vi "固定站质控流程参数读取对话框.vi"(11 "标题":string="质控流程读写") -> ()   [LabVIEW 2016, in "质控单元.lvlib"]
uses:
  <vilib>/Utility/miscctls.llb/LVPointTypeDef.ctl
panel:
  out "流程写入U16":u16[](array[numeric])
  out "退出中间":bool=TRUE
  in  "站号":enum16{"", "氨氮", "总磷", "总氮", "CODMn", "CODCr"}(ring)
  out "排液流程":u16[](array[numeric])
  out "加标流程":u16[](array[numeric])
  out "水样流程":u16[](array[numeric])
  in  "流程保存到电脑":bool
  in  "从电脑读取流程":bool
  in  "步骤10枚举":enum16{"加标", "进样", "排液", "搅拌", "定量"}(ring)
  in  "步骤10参数":dbl
  in  "步骤9枚举":enum16{"加标", "进样", "排液", "搅拌", "定量"}(ring)
  in  "步骤9参数":dbl
  in  "步骤8枚举":enum16{"加标", "进样", "排液", "搅拌", "定量"}(ring)
  in  "步骤8参数":dbl
  in  "步骤7枚举":enum16{"加标", "进样", "排液", "搅拌", "定量"}(ring)
  in  "步骤7参数":dbl
  in  "步骤6枚举":enum16{"加标", "进样", "排液", "搅拌", "定量"}(ring)
  in  "步骤6参数":dbl
  in  "步骤5枚举":enum16{"加标", "进样", "排液", "搅拌", "定量"}(ring)
  in  "步骤5参数":dbl
  in  "步骤4枚举":enum16{"加标", "进样", "排液", "搅拌", "定量"}(ring)
  in  "步骤4参数":dbl
  in  "步骤3枚举":enum16{"加标", "进样", "排液", "搅拌", "定量"}(ring)
  in  "步骤3参数":dbl
  in  "步骤2枚举":enum16{"加标", "进样", "排液", "搅拌", "定量"}(ring)
  in  "步骤2参数":dbl
  in  "步骤1枚举":enum16{"加标", "进样", "排液", "搅拌", "定量"}(ring)
  in  "步骤1参数":dbl
  in  "小流程":u16(ring) items=["润洗", "进样"]
  in  "大流程":enum16{"水样流程", "加标流程", "排液流程"}(ring)
  in  "退出":bool
  in  "流程写入到设备":bool
  in  "从设备读取流程":bool
  # "步骤1"
  # "秒/毫升"
  # "步骤2"
  # "秒/毫升"
  # "步骤3"
  # "秒/毫升"
  # "步骤4"
  # "秒/毫升"
  # "步骤5"
  # "秒/毫升"
  # "步骤6"
  # "秒/毫升"
  # "步骤7"
  # "秒/毫升"
  # "步骤8"
  # "秒/毫升"
  # "步骤9"
  # "秒/毫升"
  # "步骤10"
  # "秒/毫升"
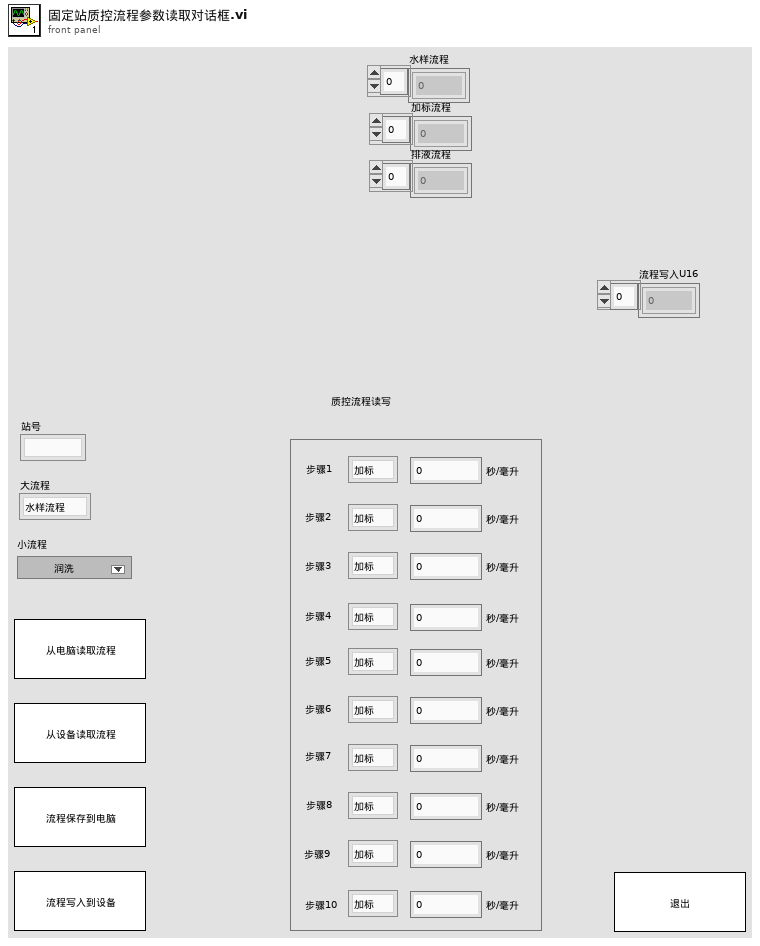
[diagram p1: front panel]
types:
  T1 = typedef "LVPointTypeDef.ctl" = cluster{"Horizontal":i16, "Vertical":i16}
  T2 = cluster{"flow1":cluster{"Type":u16, "Value":sgl}[], "flow2":cluster{"Type":u16, "Value":sgl}[], "flow3":cluster{"Type":u16, "Value":sgl}[]}
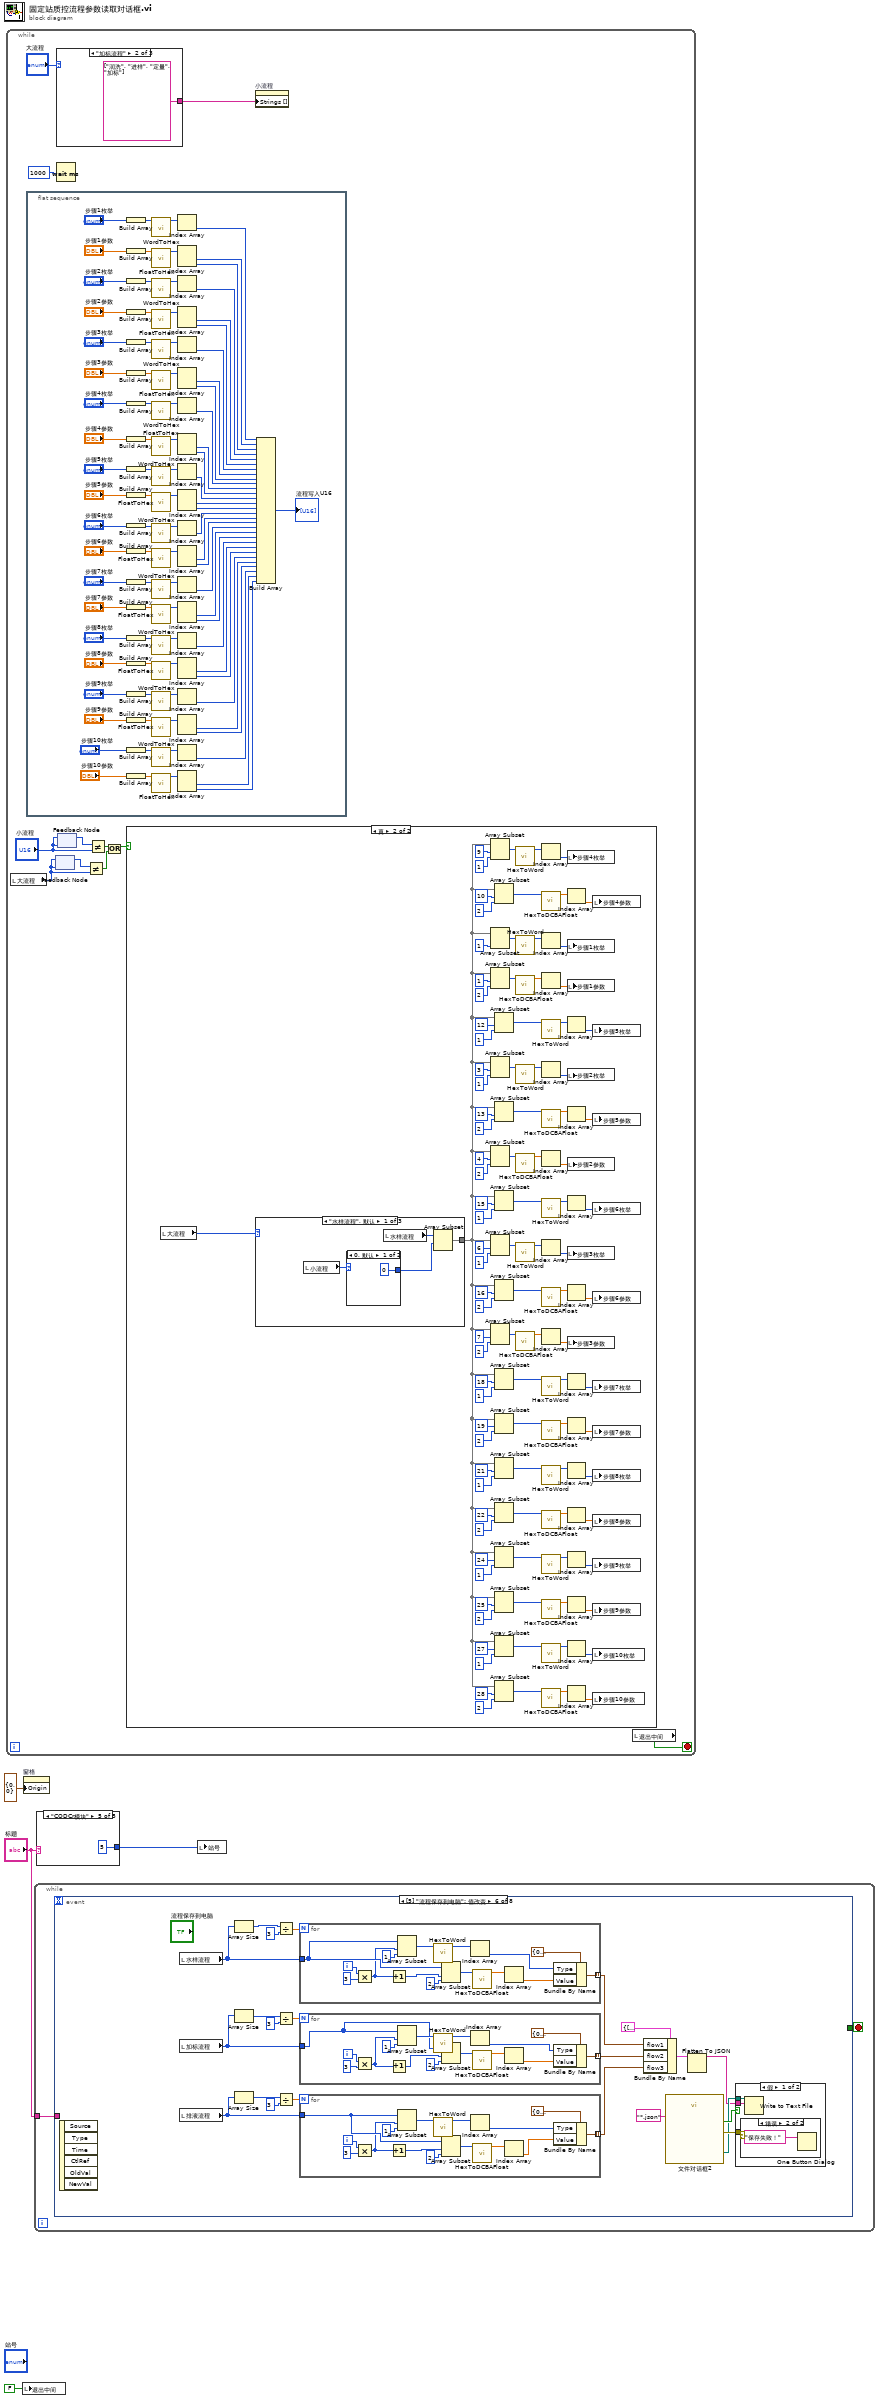
[diagram p0: block diagram]
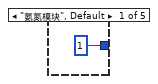
[diagram p2: hidden frame]
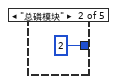
[diagram p3: hidden frame]
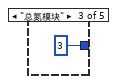
[diagram p4: hidden frame]
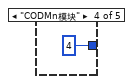
[diagram p5: hidden frame]
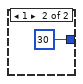
[diagram p7: hidden frame]
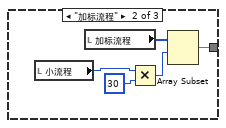
[diagram p8: hidden frame]
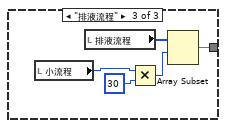
[diagram p9: hidden frame]
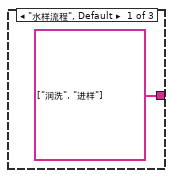
[diagram p10: hidden frame]
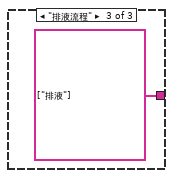
[diagram p11: hidden frame]
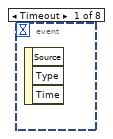
[diagram p12: hidden frame]
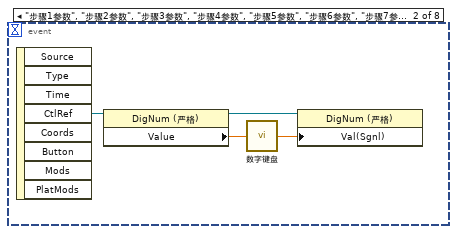
[diagram p13: hidden frame]
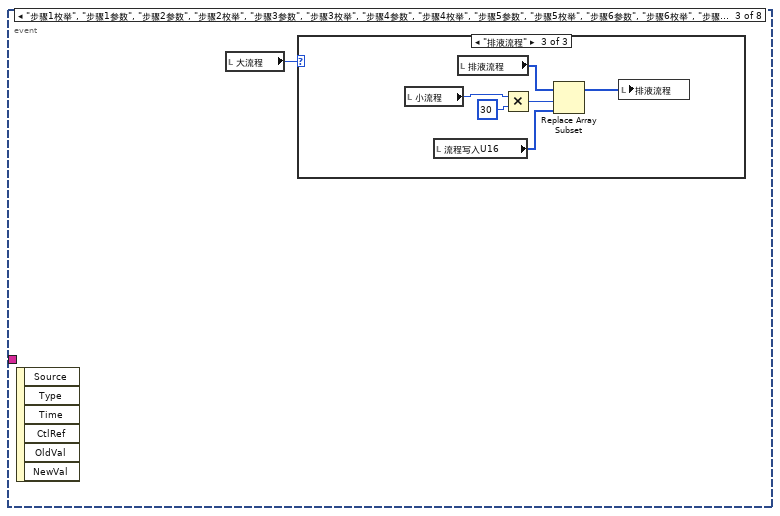
[diagram p14: hidden frame]
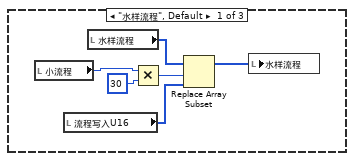
[diagram p15: hidden frame]
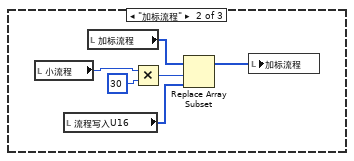
[diagram p16: hidden frame]
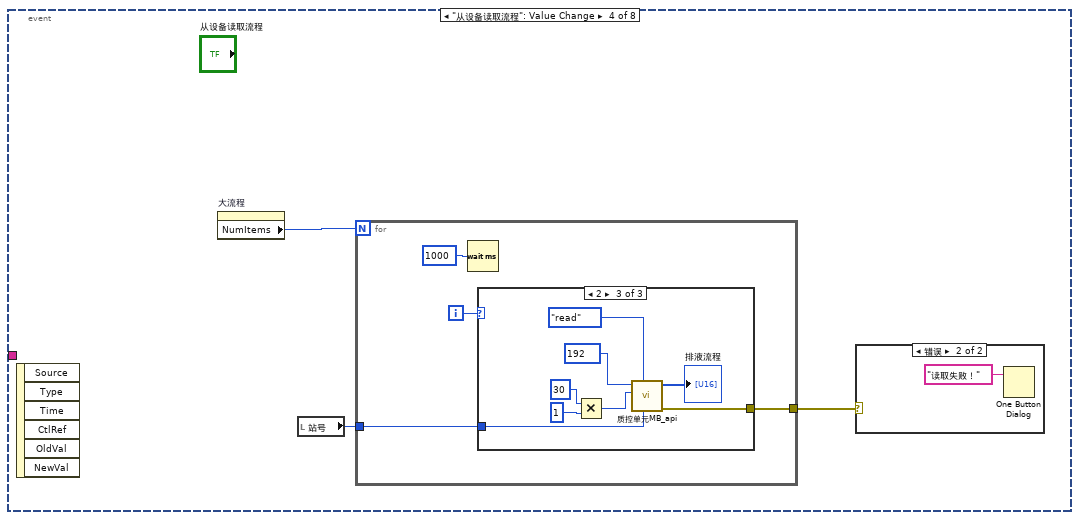
[diagram p17: hidden frame]
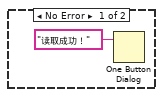
[diagram p18: hidden frame]
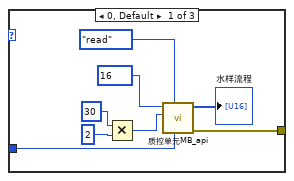
[diagram p19: hidden frame]
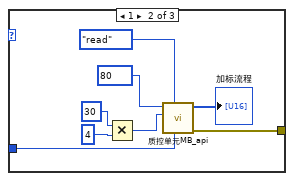
[diagram p20: hidden frame]
diagram:
  n1 = while {
    stop <- w15 stop-if-true
    n2 = local read "大流程"() -> (w5:enum16{"水样流程", "加标流程", "排液流程"})
    n3 = flat-sequence {
      frame #0 {
        n4 = Build Array("步骤1枚举") -> (w106:enum16{"加标", "进样", "排液", "搅拌", "定量"}[])
        n5 = Build Array("步骤1参数") -> (w105:dbl[])
        n6 = Build Array("步骤2枚举") -> (w100:enum16{"加标", "进样", "排液", "搅拌", "定量"}[])
        n7 = Build Array("步骤2参数") -> (w99:dbl[])
        n8 = Build Array("步骤3枚举") -> (w96:enum16{"加标", "进样", "排液", "搅拌", "定量"}[])
        n9 = Build Array("步骤3参数") -> (w95:dbl[])
        n10 = Build Array("步骤4枚举") -> (w93:enum16{"加标", "进样", "排液", "搅拌", "定量"}[])
        n11 = Build Array("步骤4参数") -> (w94:dbl[])
        n12 = Build Array("步骤5枚举") -> (w88:enum16{"加标", "进样", "排液", "搅拌", "定量"}[])
        n13 = Build Array("步骤5参数") -> (w87:dbl[])
        n14 = Build Array("步骤6枚举") -> (w85:enum16{"加标", "进样", "排液", "搅拌", "定量"}[])
        n15 = Build Array("步骤6参数") -> (w86:dbl[])
        n16 = Build Array("步骤7枚举") -> (w80:enum16{"加标", "进样", "排液", "搅拌", "定量"}[])
        n17 = Build Array("步骤7参数") -> (w79:dbl[])
        n18 = Build Array("步骤8枚举") -> (w77:enum16{"加标", "进样", "排液", "搅拌", "定量"}[])
        n19 = Build Array("步骤8参数") -> (w78:dbl[])
        n20 = Build Array("步骤9枚举") -> (w72:enum16{"加标", "进样", "排液", "搅拌", "定量"}[])
        n21 = Build Array("步骤9参数") -> (w71:dbl[])
        n22 = Build Array("步骤10枚举") -> (w69:enum16{"加标", "进样", "排液", "搅拌", "定量"}[])
        n23 = Build Array("步骤10参数") -> (w70:dbl[])
        n24 = call "WordToHex.vi"("WORD"=w106) -> ("数组"=w104:u16[])  [unwired: 10 in]
        n25 = call "FloatToHex.vi"("浮点数"=w105) -> ("DCBA整形输出"=w103:u16[])  [unwired: 10 in]
        n26 = call "WordToHex.vi"("WORD"=w100) -> ("数组"=w101:u16[])  [unwired: 10 in]
        n27 = call "FloatToHex.vi"("浮点数"=w99) -> ("DCBA整形输出"=w102:u16[])  [unwired: 10 in]
        n28 = call "WordToHex.vi"("WORD"=w96) -> ("数组"=w98:u16[])  [unwired: 10 in]
        n29 = call "FloatToHex.vi"("浮点数"=w95) -> ("DCBA整形输出"=w97:u16[])  [unwired: 10 in]
        n30 = call "WordToHex.vi"("WORD"=w93) -> ("数组"=w91:u16[])  [unwired: 10 in]
        n31 = call "FloatToHex.vi"("浮点数"=w94) -> ("DCBA整形输出"=w92:u16[])  [unwired: 10 in]
        n32 = call "WordToHex.vi"("WORD"=w88) -> ("数组"=w90:u16[])  [unwired: 10 in]
        n33 = call "FloatToHex.vi"("浮点数"=w87) -> ("DCBA整形输出"=w89:u16[])  [unwired: 10 in]
        n34 = call "WordToHex.vi"("WORD"=w85) -> ("数组"=w83:u16[])  [unwired: 10 in]
        n35 = call "FloatToHex.vi"("浮点数"=w86) -> ("DCBA整形输出"=w84:u16[])  [unwired: 10 in]
        n36 = call "WordToHex.vi"("WORD"=w80) -> ("数组"=w82:u16[])  [unwired: 10 in]
        n37 = call "FloatToHex.vi"("浮点数"=w79) -> ("DCBA整形输出"=w81:u16[])  [unwired: 10 in]
        n38 = call "WordToHex.vi"("WORD"=w77) -> ("数组"=w75:u16[])  [unwired: 10 in]
        n39 = call "FloatToHex.vi"("浮点数"=w78) -> ("DCBA整形输出"=w76:u16[])  [unwired: 10 in]
        n40 = call "WordToHex.vi"("WORD"=w72) -> ("数组"=w74:u16[])  [unwired: 10 in]
        n41 = call "FloatToHex.vi"("浮点数"=w71) -> ("DCBA整形输出"=w73:u16[])  [unwired: 10 in]
        n42 = call "WordToHex.vi"("WORD"=w69) -> ("数组"=w67:u16[])  [unwired: 10 in]
        n43 = call "FloatToHex.vi"("浮点数"=w70) -> ("DCBA整形输出"=w68:u16[])  [unwired: 10 in]
        n44 = Index Array(array=w104) -> (element=w66:u16)  [unwired: 1 in]
        n45 = Index Array(array=w103) -> (element #1=w65:u16, element #2=w64:u16)  [unwired: 2 in]
        n46 = Index Array(array=w101) -> (element=w63:u16)  [unwired: 1 in]
        n47 = Index Array(array=w102) -> (element #1=w62:u16, element #2=w61:u16)  [unwired: 2 in]
        n48 = Index Array(array=w98) -> (element=w60:u16)  [unwired: 1 in]
        n49 = Index Array(array=w97) -> (element #1=w59:u16, element #2=w58:u16)  [unwired: 2 in]
        n50 = Index Array(array=w91) -> (element=w57:u16)  [unwired: 1 in]
        n51 = Index Array(array=w92) -> (element #1=w56:u16, element #2=w55:u16)  [unwired: 2 in]
        n52 = Index Array(array=w90) -> (element=w54:u16)  [unwired: 1 in]
        n53 = Index Array(array=w89) -> (element #1=w53:u16, element #2=w52:u16)  [unwired: 2 in]
        n54 = Index Array(array=w83) -> (element=w51:u16)  [unwired: 1 in]
        n55 = Index Array(array=w84) -> (element #1=w50:u16, element #2=w49:u16)  [unwired: 2 in]
        n56 = Index Array(array=w82) -> (element=w48:u16)  [unwired: 1 in]
        n57 = Index Array(array=w81) -> (element #1=w47:u16, element #2=w46:u16)  [unwired: 2 in]
        n58 = Index Array(array=w75) -> (element=w45:u16)  [unwired: 1 in]
        n59 = Index Array(array=w76) -> (element #1=w44:u16, element #2=w43:u16)  [unwired: 2 in]
        n60 = Index Array(array=w74) -> (element=w42:u16)  [unwired: 1 in]
        n61 = Index Array(array=w73) -> (element #1=w41:u16, element #2=w40:u16)  [unwired: 2 in]
        n62 = Index Array(array=w67) -> (element=w39:u16)  [unwired: 1 in]
        n63 = Index Array(array=w68) -> (element #1=w37:u16, element #2=w38:u16)  [unwired: 2 in]
        n64 = Build Array(w66, w65, w64, w63, w62, w61, w60, w59, w58, w57, w56, w55, w54, w53, w52, w51, w50, w49, w48, w47, w46, w45, w44, w43, w42, w41, w40, w39, w37, w38) -> (→"流程写入U16":u16[])
      }
    }
    n65 = feedback #1(w5) -> (w7:enum16{"水样流程", "加标流程", "排液流程"})
    n66 = feedback-in #1(w5) -> ()
    n67 = case shown="\"加标流程\"" "大流程" {
      tunnel: [string[] ["润洗", "进样"] ("字符串[]") string[] ["润洗", "进样", "定量", "加标"] ("字符串[]") string[] ["排液"] ("字符串[]")] -> w13
      frame "水样流程", Default {
      }
      frame "加标流程" {
      }
      frame "排液流程" {
      }
    }
    n68 = Wait (ms)(milliseconds to wait=u32 1000 ("等待时间（毫秒）")) -> ()  [unwired: 1 out]
    n69 = feedback-in #2("小流程") -> ()
    n70 = feedback #2("小流程") -> (w10:u16)
    n71 = Not Equal?(x=w7, y=w5) -> (x != y?=w6:bool)
    n72 = Not Equal?(x=w10, y="小流程") -> (x != y?=w12:bool)
    n73 = Or(x=w12, y=w6) -> (x .or. y?=w8:bool)
    n74 = case shown="真" w8 {
      frame False {
      }
      frame True {
        n75 = local read "大流程"() -> (w207:enum16{"水样流程", "加标流程", "排液流程"})
        n76 = case shown="\"水样流程\", 默认" w207 {
          tunnel: [w208 w214 w219] -> w206
          frame "水样流程", Default {
            n77 = local read "小流程"() -> (w211:u16)
            n78 = case shown="0, 默认" w211 {
              tunnel: [0 ("索引") 30 ("索引")] -> w209
              frame 0, Default {
              }
              frame 1 {
              }
            }
            n79 = local read "水样流程"() -> (w210:u16[])
            n80 = Array Subset(array=w210, index=w209) -> (w208:u16[])  [unwired: 1 in]
          }
          frame "加标流程" {
            n81 = local read "小流程"() -> (w217:u16)
            n82 = local read "加标流程"() -> (w216:u16[])
            n83 = Multiply(x=w217, y=u16 30) -> (x*y=w215:u16)
            n84 = Array Subset(array=w216, index=w215) -> (w214:u16[])  [unwired: 1 in]
          }
          frame "排液流程" {
            n85 = local read "小流程"() -> (w222:u16)
            n86 = local read "排液流程"() -> (w221:u16[])
            n87 = Multiply(x=w222, y=u16 30) -> (x*y=w220:u16)
            n88 = Array Subset(array=w221, index=w220) -> (w219:u16[])  [unwired: 1 in]
          }
        }
        n89 = Array Subset(array=w206, index=9 ("索引"), length=1 ("长度")) -> (w135:u16[])
        n90 = Array Subset(array=w206, length=1 ("长度")) -> (w107:u16[])  [unwired: 1 in]
        n91 = Array Subset(array=w206, index=1 ("索引"), length=2 ("长度")) -> (w111:u16[])
        n92 = Array Subset(array=w206, index=3 ("索引"), length=1 ("长度")) -> (w123:u16[])
        n93 = Array Subset(array=w206, index=4 ("索引"), length=2 ("长度")) -> (w120:u16[])
        n94 = Array Subset(array=w206, index=6 ("索引"), length=1 ("长度")) -> (w126:u16[])
        n95 = Array Subset(array=w206, index=7 ("索引"), length=2 ("长度")) -> (w129:u16[])
        n96 = Array Subset(array=w206, index=10 ("索引"), length=2 ("长度")) -> (w138:u16[])
        n97 = Array Subset(array=w206, index=12 ("索引"), length=1 ("长度")) -> (w150:u16[])
        n98 = Array Subset(array=w206, index=13 ("索引"), length=2 ("长度")) -> (w147:u16[])
        n99 = Array Subset(array=w206, index=15 ("索引"), length=1 ("长度")) -> (w153:u16[])
        n100 = Array Subset(array=w206, index=16 ("索引"), length=2 ("长度")) -> (w156:u16[])
        n101 = Array Subset(array=w206, index=18 ("索引"), length=1 ("长度")) -> (w168:u16[])
        n102 = Array Subset(array=w206, index=19 ("索引"), length=2 ("长度")) -> (w165:u16[])
        n103 = Array Subset(array=w206, index=21 ("索引"), length=1 ("长度")) -> (w189:u16[])
        n104 = Array Subset(array=w206, index=22 ("索引"), length=2 ("长度")) -> (w192:u16[])
        n105 = Array Subset(array=w206, index=24 ("索引"), length=1 ("长度")) -> (w186:u16[])
        n106 = Array Subset(array=w206, index=25 ("索引"), length=2 ("长度")) -> (w183:u16[])
        n107 = Array Subset(array=w206, index=27 ("索引"), length=1 ("长度")) -> (w171:u16[])
        n108 = Array Subset(array=w206, index=28 ("索引"), length=2 ("长度")) -> (w174:u16[])
        n109 = call "HexToWord.vi"("数组"=w135) -> ("WORD"=w139:u16[])  [unwired: 10 in]
        n110 = call "HexToWord.vi"("数组"=w107) -> ("WORD"=w112:u16[])  [unwired: 10 in]
        n111 = call "HexToDCBAFloat.vi"("数组"=w111) -> ("FLOAT"=w113:sgl[])  [unwired: 10 in]
        n112 = call "HexToWord.vi"("数组"=w123) -> ("WORD"=w119:u16[])  [unwired: 10 in]
        n113 = call "HexToDCBAFloat.vi"("数组"=w120) -> ("FLOAT"=w118:sgl[])  [unwired: 10 in]
        n114 = call "HexToWord.vi"("数组"=w126) -> ("WORD"=w130:u16[])  [unwired: 10 in]
        n115 = call "HexToDCBAFloat.vi"("数组"=w129) -> ("FLOAT"=w131:sgl[])  [unwired: 10 in]
        n116 = Index Array(array=w139) -> (element=w142:u16)  [unwired: 1 in]
        n117 = call "HexToDCBAFloat.vi"("数组"=w138) -> ("FLOAT"=w140:sgl[])  [unwired: 10 in]
        n118 = Index Array(array=w112) -> (element=w115:u16)  [unwired: 1 in]
        n119 = Index Array(array=w113) -> (element=w114:sgl)  [unwired: 1 in]
        n120 = call "HexToWord.vi"("数组"=w150) -> ("WORD"=w146:u16[])  [unwired: 10 in]
        n121 = Index Array(array=w119) -> (element=w116:u16)  [unwired: 1 in]
        n122 = call "HexToDCBAFloat.vi"("数组"=w147) -> ("FLOAT"=w145:sgl[])  [unwired: 10 in]
        n123 = Index Array(array=w118) -> (element=w117:sgl)  [unwired: 1 in]
        n124 = call "HexToWord.vi"("数组"=w153) -> ("WORD"=w157:u16[])  [unwired: 10 in]
        n125 = Index Array(array=w130) -> (element=w133:u16)  [unwired: 1 in]
        n126 = call "HexToDCBAFloat.vi"("数组"=w156) -> ("FLOAT"=w158:sgl[])  [unwired: 10 in]
        n127 = Index Array(array=w131) -> (element=w132:sgl)  [unwired: 1 in]
        n128 = call "HexToWord.vi"("数组"=w168) -> ("WORD"=w164:u16[])  [unwired: 10 in]
        n129 = call "HexToDCBAFloat.vi"("数组"=w165) -> ("FLOAT"=w163:sgl[])  [unwired: 10 in]
        n130 = call "HexToWord.vi"("数组"=w189) -> ("WORD"=w193:u16[])  [unwired: 10 in]
        n131 = call "HexToDCBAFloat.vi"("数组"=w192) -> ("FLOAT"=w194:sgl[])  [unwired: 10 in]
        n132 = call "HexToWord.vi"("数组"=w186) -> ("WORD"=w182:u16[])  [unwired: 10 in]
        n133 = call "HexToDCBAFloat.vi"("数组"=w183) -> ("FLOAT"=w181:sgl[])  [unwired: 10 in]
        n134 = call "HexToWord.vi"("数组"=w171) -> ("WORD"=w175:u16[])  [unwired: 10 in]
        n135 = call "HexToDCBAFloat.vi"("数组"=w174) -> ("FLOAT"=w176:sgl[])  [unwired: 10 in]
        n136 = local write "步骤4枚举"(w142) -> ()
        n137 = Index Array(array=w140) -> (element=w141:sgl)  [unwired: 1 in]
        n138 = local write "步骤1枚举"(w115) -> ()
        n139 = local write "步骤1参数"(w114) -> ()
        n140 = Index Array(array=w146) -> (element=w143:u16)  [unwired: 1 in]
        n141 = local write "步骤2枚举"(w116) -> ()
        n142 = Index Array(array=w145) -> (element=w144:sgl)  [unwired: 1 in]
        n143 = local write "步骤2参数"(w117) -> ()
        n144 = Index Array(array=w157) -> (element=w160:u16)  [unwired: 1 in]
        n145 = local write "步骤3枚举"(w133) -> ()
        n146 = Index Array(array=w158) -> (element=w159:sgl)  [unwired: 1 in]
        n147 = local write "步骤3参数"(w132) -> ()
        n148 = Index Array(array=w164) -> (element=w161:u16)  [unwired: 1 in]
        n149 = Index Array(array=w163) -> (element=w162:sgl)  [unwired: 1 in]
        n150 = Index Array(array=w193) -> (element=w196:u16)  [unwired: 1 in]
        n151 = Index Array(array=w194) -> (element=w195:sgl)  [unwired: 1 in]
        n152 = Index Array(array=w182) -> (element=w179:u16)  [unwired: 1 in]
        n153 = Index Array(array=w181) -> (element=w180:sgl)  [unwired: 1 in]
        n154 = Index Array(array=w175) -> (element=w178:u16)  [unwired: 1 in]
        n155 = Index Array(array=w176) -> (element=w177:sgl)  [unwired: 1 in]
        n156 = local write "步骤4参数"(w141) -> ()
        n157 = local write "步骤5枚举"(w143) -> ()
        n158 = local write "步骤5参数"(w144) -> ()
        n159 = local write "步骤6枚举"(w160) -> ()
        n160 = local write "步骤6参数"(w159) -> ()
        n161 = local write "步骤7枚举"(w161) -> ()
        n162 = local write "步骤7参数"(w162) -> ()
        n163 = local write "步骤8枚举"(w196) -> ()
        n164 = local write "步骤8参数"(w195) -> ()
        n165 = local write "步骤9枚举"(w179) -> ()
        n166 = local write "步骤9参数"(w180) -> ()
        n167 = local write "步骤10枚举"(w178) -> ()
        n168 = local write "步骤10参数"(w177) -> ()
      }
    }
    n169 = property on="小流程" class="Ring (严格)"("Strings []"=w13) -> ()  [unwired: 2 in, 2 out]
    n170 = local read "退出中间"() -> (w15:bool)
  }
  n171 = local write "退出中间"(FALSE ("退出中间")) -> ()
  n172 = property on="窗格" class="Pane"("Origin"=T1 {"Horizontal"=0, "Vertical"=0} ("原点")) -> ()  [unwired: 2 in, 2 out]
  n173 = while {
    tunnel: "标题" -> [w228]
    stop <- w227 stop-if-true
    n174 = event shown="[5] \"流程保存到电脑\": 值改变" {
      selector: _ -> [_ _ _ _ _ _ _ _]
      dyn-events: _ -> [_ _ _ _ _ _ _ _]
      timeout: _ -> [_ _ _ _ _ _ _ _]
      tunnel: w228 -> [_ _ _ _ _ _ w406 _]
      tunnel: [_ _ _ _ _ _ _ w420] -> w227
      event Timeout {
        n175 = event-data() -> ()  [unwired: 1 in, 3 out]
      }
      event "步骤1参数", "步骤2参数", "步骤3参数", "步骤4参数", "步骤5参数", "步骤6参数", "步骤7参数", "步骤8参数", "步骤9参数", "步骤10参数": Mouse Down {
        n176 = event-data() -> ("CtlRef"=w232:refnum<vi>)  [unwired: 1 in, 7 out]
        n177 = property class="DigNum (严格)"(reference=w232) -> (reference out=w231:refnum<vi>, "Value"=w230:dbl)  [unwired: 1 in, 1 out]
        n178 = call "数字键盘.vi"("OldNumber"=w230) -> ("NewNumber"=w229:sgl)
        n179 = property class="DigNum (严格)"(reference=w231, "Val(Sgnl)"=w229) -> ()  [unwired: 1 in, 2 out]
      }
      event "步骤1枚举", "步骤1参数", "步骤2参数", "步骤2枚举", "步骤3参数", "步骤3枚举", "步骤4参数", "步骤4枚举", "步骤5参数", "步骤5枚举", "步骤6参数", "步骤6枚举", "步骤7参数", "步骤7枚举", "步骤8参数", "步骤8枚举", "步骤9参数", "步骤9枚举", "步骤10参数", "步骤10枚举": Value Change {
        n180 = event-data() -> ()  [unwired: 1 in, 6 out]
        n181 = local read "大流程"() -> (w233:enum16{"水样流程", "加标流程", "排液流程"})
        n182 = case shown="\"排液流程\"" w233 {
          frame "水样流程", Default {
            n183 = local read "小流程"() -> (w239:u16)
            n184 = local read "流程写入U16"() -> (w235:u16[])
            n185 = local read "水样流程"() -> (w237:u16[])
            n186 = Multiply(x=w239, y=u16 30) -> (x*y=w236:u16)
            n187 = Replace Array Subset(array=w237, new element=w235, index=w236) -> (w234:u16[])
            n188 = local write "水样流程"(w234) -> ()
          }
          frame "加标流程" {
            n189 = local read "小流程"() -> (w245:u16)
            n190 = local read "流程写入U16"() -> (w241:u16[])
            n191 = local read "加标流程"() -> (w243:u16[])
            n192 = Multiply(x=w245, y=u16 30) -> (x*y=w242:u16)
            n193 = Replace Array Subset(array=w243, new element=w241, index=w242) -> (w240:u16[])
            n194 = local write "加标流程"(w240) -> ()
          }
          frame "排液流程" {
            n195 = local read "小流程"() -> (w251:u16)
            n196 = local read "流程写入U16"() -> (w247:u16[])
            n197 = local read "排液流程"() -> (w249:u16[])
            n198 = Multiply(x=w251, y=u16 30) -> (x*y=w248:u16)
            n199 = Replace Array Subset(array=w249, new element=w247, index=w248) -> (w246:u16[])
            n200 = local write "排液流程"(w246) -> ()
          }
        }
      }
      event "从设备读取流程": Value Change {
        n201 = event-data() -> ()  [unwired: 1 in, 6 out]
        n202 = property on="大流程" class="Enum (严格)"() -> ("NumItems"=w254:u32)  [unwired: 2 in, 2 out]
        n203 = local read "站号"() -> (w252:enum16{"", "氨氮", "总磷", "总氮", "CODMn", "CODCr"})
        n204 = for {
          N: w254 -> [_]
          tunnel: [w259] -> w253
          tunnel: w252 -> [w258]
          i -> [w260]
          n205 = Wait (ms)(milliseconds to wait=u32 1000 ("等待时间（毫秒）")) -> ()  [unwired: 1 out]
          n206 = case shown="2" w260 {
            tunnel: [w262 w270 w278] -> w259
            tunnel: w258 -> [w261 w269 w277]
            frame 0, Default {
              n207 = Multiply(x=u32 30, y=u32 2) -> (x*y=w264:u32)
              n208 = call "质控单元MB_api.vi"("Slave ID"=w261, "STEP"=enum16{"open", "read", "write", "close"}."read", "quantity"=w264, "starting address"=u16 16) -> ("error out"=w262:errorcluster, "Registers"=→"水样流程":u16[])  [unwired: 5 in, 1 out]
            }
            frame 1 {
              n209 = Multiply(x=u32 30, y=u32 4) -> (x*y=w272:u32)
              n210 = call "质控单元MB_api.vi"("Slave ID"=w269, "STEP"=enum16{"open", "read", "write", "close"}."read", "quantity"=w272, "starting address"=u16 80) -> ("error out"=w270:errorcluster, "Registers"=→"加标流程":u16[])  [unwired: 5 in, 1 out]
            }
            frame 2 {
              n211 = Multiply(x=u32 30, y=u32 1) -> (x*y=w280:u32)
              n212 = call "质控单元MB_api.vi"("Slave ID"=w277, "STEP"=enum16{"open", "read", "write", "close"}."read", "quantity"=w280, "starting address"=u16 192) -> ("error out"=w278:errorcluster, "Registers"=→"排液流程":u16[])  [unwired: 5 in, 1 out]
            }
          }
        }
        n213 = case shown="错误" w253 {
          frame No Error {
            n214 = One Button Dialog(message="读取成功！" ("消息")) -> ()  [unwired: 1 in, 1 out]
          }
          frame Error {
            n215 = One Button Dialog(message="读取失败！" ("消息")) -> ()  [unwired: 1 in, 1 out]
          }
        }
      }
      event "从电脑读取流程": Value Change {
        n216 = event-data() -> ()  [unwired: 1 in, 6 out]
        n217 = Read from Text File() -> (text=w288:string)  [unwired: 4 in, 3 out]
        n218 = Unflatten From JSON(JSON string=w288, type and defaults=T2 {"flow1"=[], "flow2"=[], "flow3"=[]}) -> (value=w286:T2, error out=w287:errorcluster)  [unwired: 5 in]
        n219 = case shown="无错误" w287 {
          tunnel: w286 -> [w296 _]
          frame No Error {
            n220 = Unbundle By Name(w296) -> ("flow1"=w295:cluster{"Type":u16, "Value":sgl}[], "flow2"=w294:cluster{"Type":u16, "Value":sgl}[], "flow3"=w293:cluster{"Type":u16, "Value":sgl}[])
            n221 = for {
              tunnel: w295 -> [w326] mode=indexing
              shift-right: [w318] -> w290
              shift-left: _ -> [w317]
              n222 = Unbundle By Name(w326) -> ("Type"=w325:u16, "Value"=w323:sgl)
              n223 = Build Array(w325) -> (w324:u16[])
              n224 = Build Array(w323) -> (w322:sgl[])
              n225 = call "WordToHex.vi"("WORD"=w324) -> ("数组"=w321:u16[])  [unwired: 10 in]
              n226 = call "FloatToHex.vi"("浮点数"=w322) -> ("DCBA整形输出"=w320:u16[])  [unwired: 10 in]
              n227 = Insert Into Array(array=w321, new element=w320) -> (w319:u16[])  [unwired: 1 in]
              n228 = Insert Into Array(array=w317, new element=w319) -> (w318:u16[])  [unwired: 1 in]
            }
            n229 = for {
              tunnel: w294 -> [w316] mode=indexing
              shift-right: [w308] -> w291
              shift-left: _ -> [w307]
              n230 = Unbundle By Name(w316) -> ("Type"=w315:u16, "Value"=w313:sgl)
              n231 = Build Array(w315) -> (w314:u16[])
              n232 = Build Array(w313) -> (w312:sgl[])
              n233 = call "WordToHex.vi"("WORD"=w314) -> ("数组"=w311:u16[])  [unwired: 10 in]
              n234 = call "FloatToHex.vi"("浮点数"=w312) -> ("DCBA整形输出"=w310:u16[])  [unwired: 10 in]
              n235 = Insert Into Array(array=w311, new element=w310) -> (w309:u16[])  [unwired: 1 in]
              n236 = Insert Into Array(array=w307, new element=w309) -> (w308:u16[])  [unwired: 1 in]
            }
            n237 = for {
              tunnel: w293 -> [w306] mode=indexing
              shift-right: [w298] -> w292
              shift-left: _ -> [w297]
              n238 = Unbundle By Name(w306) -> ("Type"=w305:u16, "Value"=w303:sgl)
              n239 = Build Array(w305) -> (w304:u16[])
              n240 = Build Array(w303) -> (w302:sgl[])
              n241 = call "WordToHex.vi"("WORD"=w304) -> ("数组"=w301:u16[])  [unwired: 10 in]
              n242 = call "FloatToHex.vi"("浮点数"=w302) -> ("DCBA整形输出"=w300:u16[])  [unwired: 10 in]
              n243 = Insert Into Array(array=w301, new element=w300) -> (w299:u16[])  [unwired: 1 in]
              n244 = Insert Into Array(array=w297, new element=w299) -> (w298:u16[])  [unwired: 1 in]
            }
            n245 = One Button Dialog(message="读取成功！" ("消息")) -> ()  [unwired: 1 in, 1 out]
            n246 = local write "水样流程"(w290) -> ()
            n247 = local write "加标流程"(w291) -> ()
            n248 = local write "排液流程"(w292) -> ()
          }
          frame Error {
            n249 = One Button Dialog(message="读取失败！" ("消息")) -> ()  [unwired: 1 in, 1 out]
          }
        }
      }
      event "流程保存到电脑": Value Change {
        n250 = event-data() -> ()  [unwired: 1 in, 6 out]
        n251 = local read "水样流程"() -> (w337:u16[])
        n252 = local read "加标流程"() -> (w340:u16[])
        n253 = local read "排液流程"() -> (w347:u16[])
        n254 = Array Size(array=w337) -> (size(s)=w334:i32)
        n255 = Array Size(array=w340) -> (size(s)=w343:i32)
        n256 = Array Size(array=w347) -> (size(s)=w344:i32)
        n257 = Divide(x=w334, y=3) -> (x/y=w336:dbl)
        n258 = Divide(x=w343, y=3) -> (x/y=w341:dbl)
        n259 = Divide(x=w344, y=3) -> (x/y=w346:dbl)
        n260 = for {
          N: w336 -> [_]
          tunnel: w337 -> [w397]
          tunnel: [w386] -> w339 mode=indexing
          i -> [w395]
          n261 = Multiply(x=w395, y=3) -> (x*y=w393:i32)
          n262 = Increment(x=w393) -> (x+1=w392:i32)
          n263 = Array Subset(array=w397, index=w393, length=1 ("长度")) -> (w400:u16[])
          n264 = call "HexToWord.vi"("数组"=w400) -> ("WORD"=w390:u16[])  [unwired: 10 in]
          n265 = Array Subset(array=w397, index=w392, length=2 ("长度")) -> (w398:u16[])
          n266 = Index Array(array=w390) -> (element=w389:u16)  [unwired: 1 in]
          n267 = call "HexToDCBAFloat.vi"("数组"=w398) -> ("FLOAT"=w388:sgl[])  [unwired: 10 in]
          n268 = Index Array(array=w388) -> (element=w387:sgl)  [unwired: 1 in]
          n269 = Bundle By Name(cluster=cluster{"Type":u16, "Value":sgl} {"Type"=0, "Value"=0.0}, "Type"=w389, "Value"=w387) -> (w386:cluster{"Type":u16, "Value":sgl})
        }
        n270 = for {
          N: w341 -> [_]
          tunnel: w340 -> [w382]
          tunnel: [w371] -> w348 mode=indexing
          i -> [w380]
          n271 = Multiply(x=w380, y=3) -> (x*y=w378:i32)
          n272 = Increment(x=w378) -> (x+1=w377:i32)
          n273 = Array Subset(array=w382, index=w378, length=1 ("长度")) -> (w385:u16[])
          n274 = call "HexToWord.vi"("数组"=w385) -> ("WORD"=w375:u16[])  [unwired: 10 in]
          n275 = Array Subset(array=w382, index=w377, length=2 ("长度")) -> (w383:u16[])
          n276 = Index Array(array=w375) -> (element=w374:u16)  [unwired: 1 in]
          n277 = call "HexToDCBAFloat.vi"("数组"=w383) -> ("FLOAT"=w373:sgl[])  [unwired: 10 in]
          n278 = Index Array(array=w373) -> (element=w372:sgl)  [unwired: 1 in]
          n279 = Bundle By Name(cluster=cluster{"Type":u16, "Value":sgl} {"Type"=0, "Value"=0.0}, "Type"=w374, "Value"=w372) -> (w371:cluster{"Type":u16, "Value":sgl})
        }
        n280 = for {
          N: w346 -> [_]
          tunnel: w347 -> [w367]
          tunnel: [w356] -> w349 mode=indexing
          i -> [w365]
          n281 = Multiply(x=w365, y=3) -> (x*y=w363:i32)
          n282 = Increment(x=w363) -> (x+1=w362:i32)
          n283 = Array Subset(array=w367, index=w363, length=1 ("长度")) -> (w370:u16[])
          n284 = call "HexToWord.vi"("数组"=w370) -> ("WORD"=w360:u16[])  [unwired: 10 in]
          n285 = Array Subset(array=w367, index=w362, length=2 ("长度")) -> (w368:u16[])
          n286 = Index Array(array=w360) -> (element=w359:u16)  [unwired: 1 in]
          n287 = call "HexToDCBAFloat.vi"("数组"=w368) -> ("FLOAT"=w358:sgl[])  [unwired: 10 in]
          n288 = Index Array(array=w358) -> (element=w357:sgl)  [unwired: 1 in]
          n289 = Bundle By Name(cluster=cluster{"Type":u16, "Value":sgl} {"Type"=0, "Value"=0.0}, "Type"=w359, "Value"=w357) -> (w356:cluster{"Type":u16, "Value":sgl})
        }
        n290 = Bundle By Name(cluster=T2 {"flow1"=[], "flow2"=[], "flow3"=[]}, "flow1"=w339, "flow2"=w348, "flow3"=w349) -> (w333:T2)
        n291 = call "文件对话框2"("pattern (all files)"="*.json") -> ("selected path"=w330:path, "cancelled"=w331:bool, "error out"=w332:errorcluster)  [unwired: 11 in, 1 out]
        n292 = Flatten To JSON(anything=w333) -> (JSON string=w328:string)  [unwired: 2 in, 1 out]
        n293 = case shown="假" w331 {
          tunnel: w330 -> [w352 _]
          tunnel: w332 -> [w350 _]
          tunnel: w328 -> [w351 _]
          frame False {
            n294 = case shown="错误" w350 {
              frame No Error {
                n295 = One Button Dialog(message="保存成功！" ("消息")) -> ()  [unwired: 1 in, 1 out]
              }
              frame Error {
                n296 = One Button Dialog(message="保存失败！" ("消息")) -> ()  [unwired: 1 in, 1 out]
              }
            }
            n297 = Write to Text File(file (use dialog)=w352, text=w351) -> ()  [unwired: 2 in, 3 out]
          }
          frame True {
            n298 = One Button Dialog(message="保存失败！" ("消息")) -> ()  [unwired: 1 in, 1 out]
          }
        }
      }
      event "流程写入到设备": Value Change {
        n299 = event-data() -> ()  [unwired: 1 in, 6 out]
        n300 = case shown="\"氨氮模块\", 默认" w406 {
          tunnel: [u8 1 ("Slave ID") u8 2 ("Slave ID") u8 3 ("Slave ID") u8 4 ("Slave ID") u8 5 ("Slave ID")] -> w405
          frame "氨氮模块", Default {
          }
          frame "总磷模块" {
          }
          frame "总氮模块" {
          }
          frame "CODMn模块" {
          }
          frame "CODCr模块" {
          }
        }
        n301 = local read "大流程"() -> (w402:enum16{"水样流程", "加标流程", "排液流程"})
        n302 = case shown="\"排液流程\"" w402 {
          tunnel: [w408 w410 w412] -> w403
          tunnel: [u16 16 ("starting address") u16 80 ("starting address") u16 192 ("starting address")] -> w401
          frame "水样流程", Default {
            n303 = local read "水样流程"() -> (w408:u16[])
          }
          frame "加标流程" {
            n304 = local read "加标流程"() -> (w410:u16[])
          }
          frame "排液流程" {
            n305 = local read "排液流程"() -> (w412:u16[])
          }
        }
        n306 = call "写入参数.vi"("values"=w403, "starting address"=w401, "Slave ID"=w405) -> ("error out"=w404:errorcluster)  [unwired: 8 in]
        n307 = case shown="错误" w404 {
          frame No Error {
            n308 = One Button Dialog(message="写入成功！" ("消息")) -> ()  [unwired: 1 in, 1 out]
          }
          frame Error {
            n309 = One Button Dialog(message="写入失败！" ("消息")) -> ()  [unwired: 1 in, 1 out]
          }
        }
      }
      event "退出": Value Change {
        w420 = TRUE
        n310 = event-data() -> ()  [unwired: 1 in, 6 out]
        "退出中间" <- w420
      }
    }
  }
  n311 = case shown="\"CODCr模块\"" "标题" {
    tunnel: [u8 1 ("Slave ID") u8 2 ("Slave ID") u8 3 ("Slave ID") u8 4 ("Slave ID") u8 5 ("Slave ID")] -> w2
    frame "氨氮模块", Default {
    }
    frame "总磷模块" {
    }
    frame "总氮模块" {
    }
    frame "CODMn模块" {
    }
    frame "CODCr模块" {
    }
  }
  n312 = local write "站号"(w2) -> ()
